vi "Read Parity.vi"(8 "error in (no error)":errorcluster, 11 "serial slave in":refnum<class "Serial Slave.lvclass">) -> (0 "error out":errorcluster, 2 "parity":u16(ring) items=["None", "Odd", "Even", "Mark", "Space"], 3 "serial slave out":refnum<class "Serial Slave.lvclass">)   [LabVIEW 2017, in "SubVIs.lvlib" / "Serial Slave.lvclass"]
uses:
  <vilib>/Modbus/subvis/Protocol/Serial/Serial Slave/Serial Slave.lvclass
  <vilib>/Modbus/subvis/Protocol/Serial/Serial Slave/Serial Slave.lvclass/Serial Slave.ctl
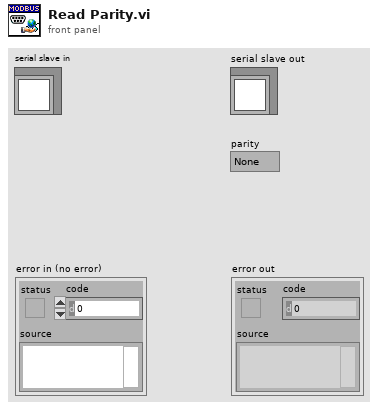
[diagram p1: front panel]
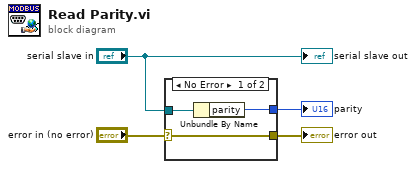
[diagram p0: block diagram]
diagram:
  n1 = case shown="No Error" "error in (no error)" {
    selector: "error in (no error)" -> [w5 w8]
    tunnel: "serial slave in" -> [w7 _]
    tunnel: [w6 _] -> w3
    tunnel: [w5 w8] -> w1
    frame No Error {
      n2 = Unbundle By Name(w7) -> ("parity"=w6:u16)
    }
    frame Error {
    }
  }
  "error out" <- w1
  "parity" <- w3
  "serial slave out" <- "serial slave in"
